vi "Remove All Sessions.vi"(8 "error in (no error)":errorcluster, 11 "connection map in":refnum<class "Connection Map.lvclass">) -> (0 "error out":errorcluster, 3 "connection map out":refnum<class "Connection Map.lvclass">)   [LabVIEW 2020, in "MeasurementLink Session Management.lvlib" / "Connection Map.lvclass"]
uses:
  Connection Map.lvclass
  Connection Map.lvclass/Connection Map.ctl
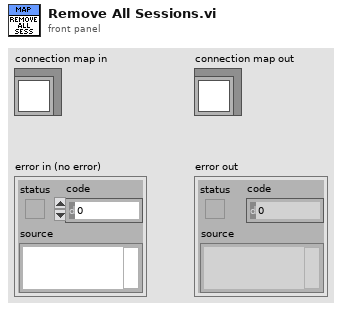
[diagram p1: front panel]
types:
  T1 = typedef "MeasurementLink Session Management.lvlib/Session Reservation.lvclass/Connection with Session.ctl" = cluster{"connection":T2, "session":variant}
  T2 = typedef "MeasurementLink Session Management.lvlib/Session Reservation.lvclass/Connection.ctl" = cluster{"pin or relay name":string, "site":i32, "instrument type id":string, "channel":string}
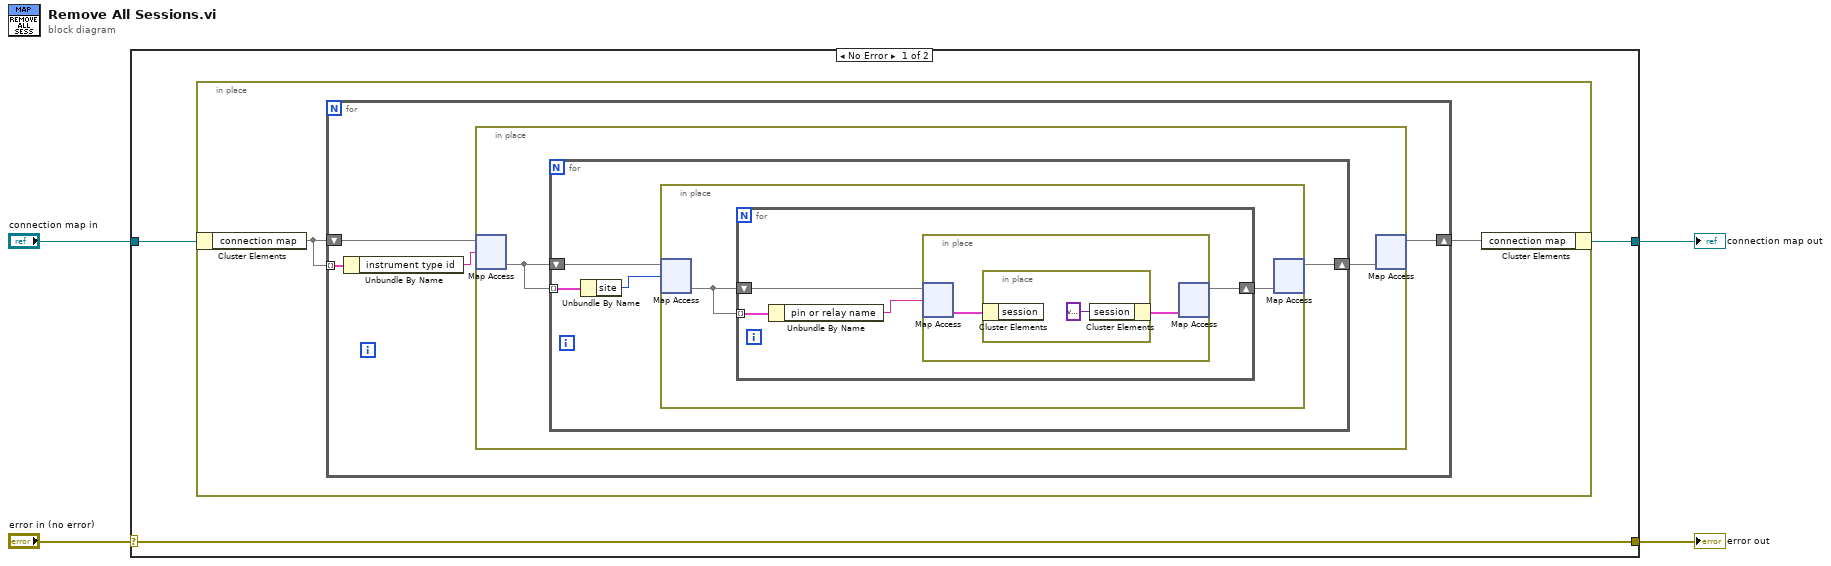
[diagram p0: block diagram]
diagram:
  n1 = case shown="No Error" "error in (no error)" {
    selector: "error in (no error)" -> [w7 w30]
    tunnel: [w7 w30] -> w3
    tunnel: [w5 w29] -> w1
    tunnel: "connection map in" -> [w6 w29]
    frame No Error {
      n2 = in-place {
        n3 = in-place-cluster #1(w6) -> ("connection map"=w9:map{string, map{i32, map{string, T1}}})
        n4 = for {
          tunnel: w9 -> [w12] mode=indexing
          shift-right: [w10] -> w8
          shift-left: w9 -> [w13]
          n5 = Unbundle By Name(w12) -> ("instrument type id"=w11:string)
          n6 = in-place {
            n7 = in-place-map #2(w13, w11) -> (w15:map{i32, map{string, T1}})  [unwired: 1 in, 1 out]
            n8 = for {
              shift-right: [w16] -> w14
              shift-left: w15 -> [w18]
              tunnel: w15 -> [w19] mode=indexing
              n9 = Unbundle By Name(w19) -> ("site"=w17:i32)
              n10 = in-place {
                n11 = in-place-map #3(w18, w17) -> (w21:map{string, T1})  [unwired: 1 in, 1 out]
                n12 = for {
                  shift-right: [w22] -> w20
                  shift-left: w21 -> [w25]
                  tunnel: w21 -> [w24] mode=indexing
                  n13 = Unbundle By Name(w24) -> ("pin or relay name"=w23:string)
                  n14 = in-place {
                    n15 = in-place-map #4(w25, w23) -> (w27:T1)  [unwired: 1 in, 1 out]
                    n16 = in-place {
                      n17 = in-place-cluster #5(w27) -> ()  [unwired: 1 out]
                      n18 = in-place-cluster #5("session"=variant) -> (w26:T1)
                    }
                    n19 = in-place-map #4(w26) -> (w22:map{string, T1})  [unwired: 1 in, 2 out]
                  }
                }
                n20 = in-place-map #3(w20) -> (w16:map{i32, map{string, T1}})  [unwired: 1 in, 2 out]
              }
            }
            n21 = in-place-map #2(w14) -> (w10:map{string, map{i32, map{string, T1}}})  [unwired: 1 in, 2 out]
          }
        }
        n22 = in-place-cluster #1("connection map"=w8) -> (w5:refnum<class "Connection Map.lvclass">)
      }
    }
    frame Error {
    }
  }
  "error out" <- w3
  "connection map out" <- w1
